vi "Keyence LJ-X8000A Read Profiles(for High Speed Data Communication).vi"() -> ()   [LabVIEW 2010]
doc: "This example mainly indicates how to acquire profiles from controllers by using <B>Read Profiles (for High-Speed Communication)</B> VI via high-speed communication."
uses:
  KEYENCE LJ-X8000A.lvlib
  Public/Clusters/Ethernet Config.ctl
  Public/Clusters/High-Speed Comm Start Req.ctl
  Public/Constants/High-Speed Comm Start Pos.ctl
  Public/Constants/High-Speed Receive Ratio.ctl
  Public/Clusters/Profile Info.ctl
panel:
  out "error out":errorcluster
  out "Comm":bool
  out "Monitoring":bool
  out "Timeout Cnt":u32
  out "Height Image":dbl[][](graph)
  out "Read Cnt":u32
  out "Notify":u32
  out "Buf Usage Rate":u32
  out "Profile Info":T1
  in  "Start Req":T2={"High-Speed Comm Start Pos"=2, "Read Profile Cnt"=1000, "High-Speed Receive Ratio"=16} {"High-Speed Receive Ratio" items=["LOWEST"=0, "LOW"=16, "MIDDLE"=17, "HIGH"=18, "HIGHEST"=32]; "High-Speed Comm Start Pos" items=["SEND COMPLETE POS", "OLDEST", "NEXT"]}
  in  "Port No":u16=24692
  in  "Stop Monitoring":bool
  in  "Start Monitoring":bool
  in  "Stop High Speed Comm":bool
  in  "Start High Speed Comm":bool
  in  "Stop VI":bool
  in  "Ethernet Config":T5={"IP Address"=[192, 168, 0, 1], "Port No"=24691}
  # "Read Profiles Start/Stop"
  # "High Speed Data Communication Start/Stop"
  # "Communication Configuration"
  # "Output from Read Profiles VI"
  # "Communication Configuration\nfor High Speed Communication"
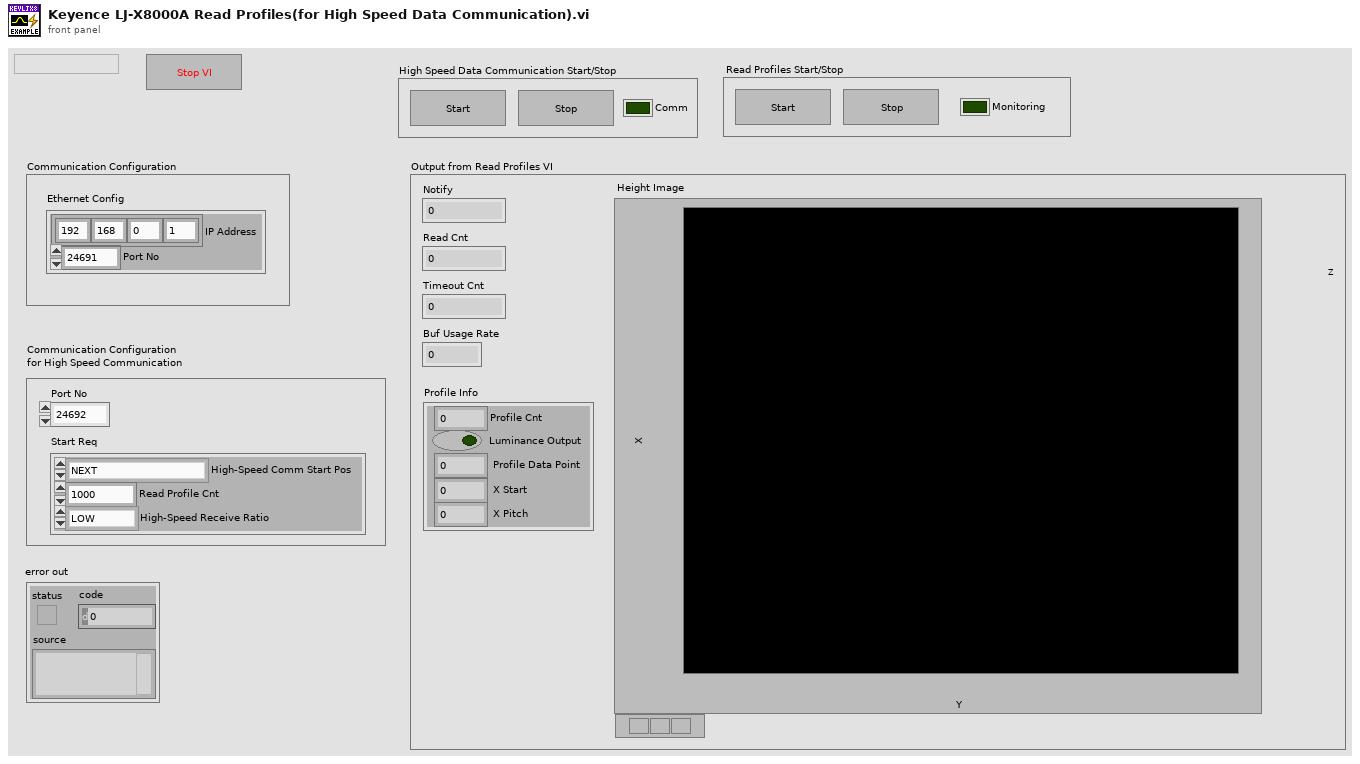
[diagram p1: front panel]
types:
  T1 = typedef "KEYENCE LJ-X8000A.lvlib/Profile Info.ctl" = cluster{"Profile Cnt":u8, "Luminance Output":bool, " Profile Data Point":u16, " X Start":i32, " X Pitch":i32}
  T2 = typedef "KEYENCE LJ-X8000A.lvlib/High-Speed Comm Start Req.ctl" = cluster{"High-Speed Comm Start Pos":T3, "Read Profile Cnt":u32, "High-Speed Receive Ratio":T4}
  T3 = typedef "KEYENCE LJ-X8000A.lvlib/High-Speed Comm Start Pos.ctl" = u8
  T4 = typedef "KEYENCE LJ-X8000A.lvlib/High-Speed Receive Ratio.ctl" = u8
  T5 = typedef "KEYENCE LJ-X8000A.lvlib/Ethernet Config.ctl" = cluster{"IP Address":u8[], "Port No":u16}
  T6 = enum8{"Enabled", "Disabled", "Disabled and Grayed Out"}
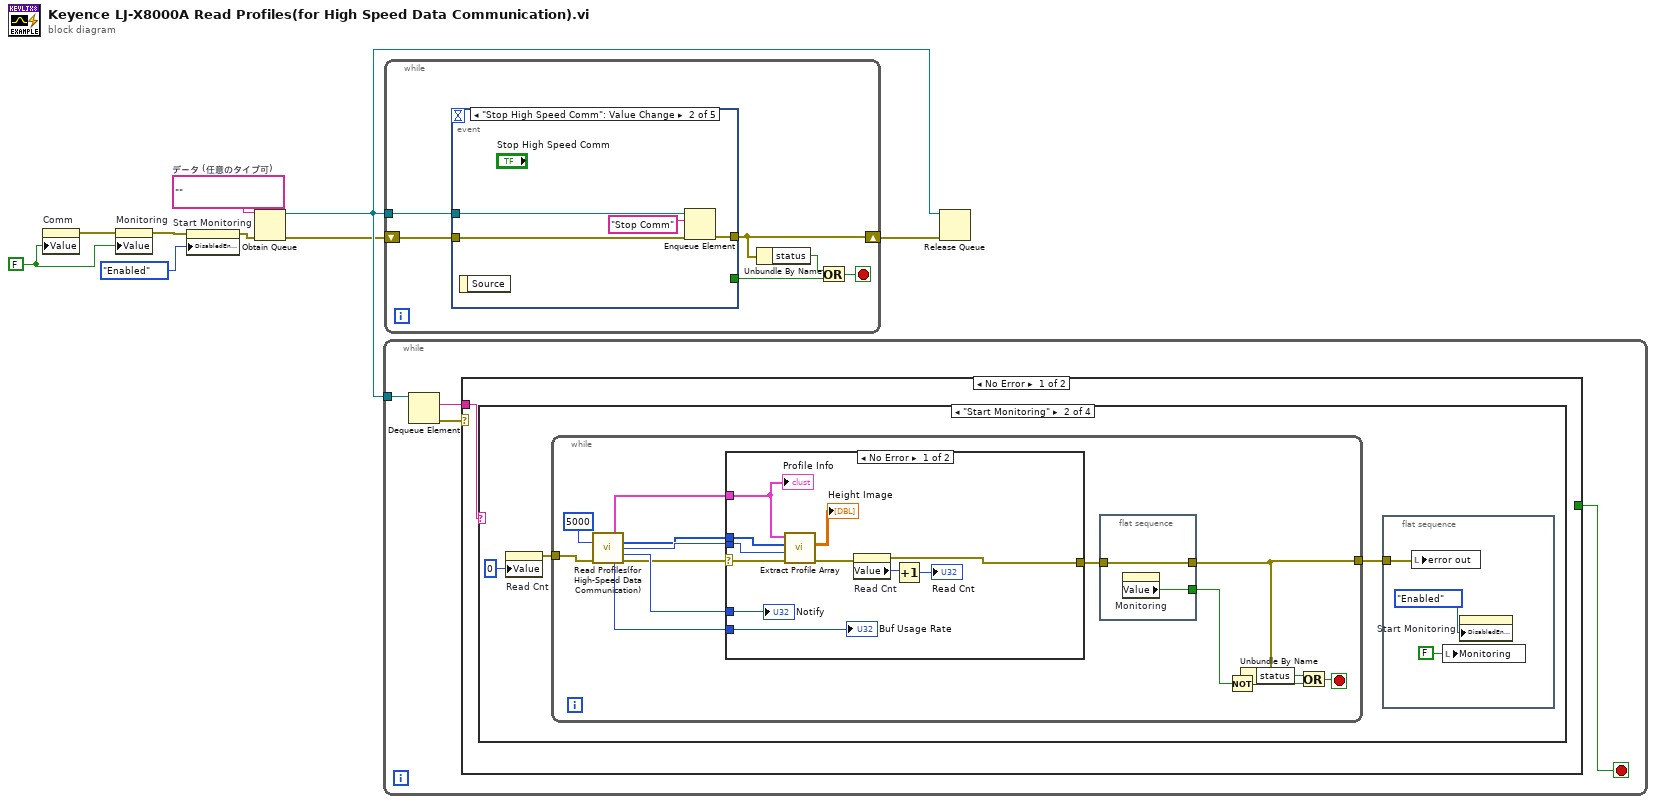
[diagram p0: block diagram]
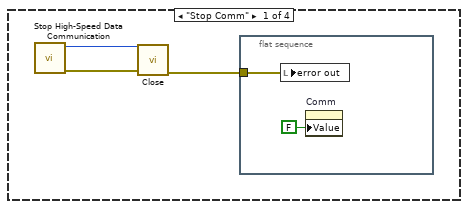
[diagram p2: hidden frame]
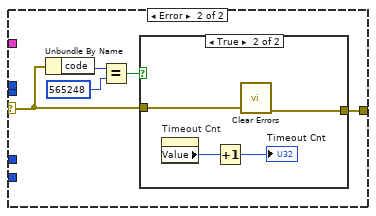
[diagram p3: hidden frame]
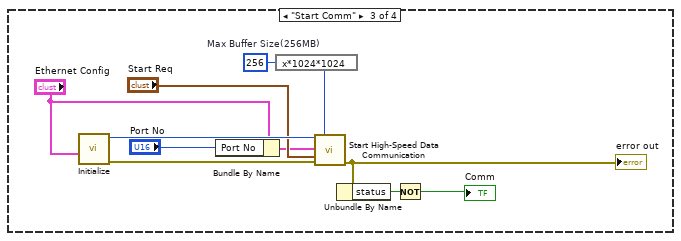
[diagram p5: hidden frame]
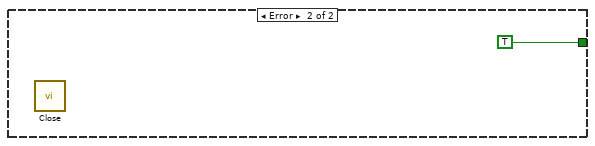
[diagram p7: hidden frame]
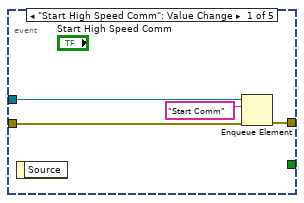
[diagram p8: hidden frame]
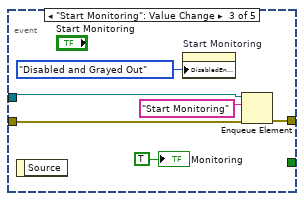
[diagram p9: hidden frame]
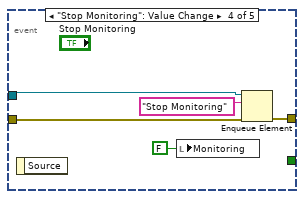
[diagram p10: hidden frame]
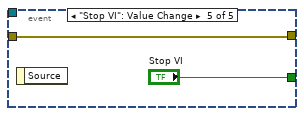
[diagram p11: hidden frame]
diagram:
  w5 = FALSE ("Monitoring")
  w7 = ""  # データ (任意のタイプ可)
  n1 = property on="Comm" class="Bool (strict)"("Value"=w5) -> (error out=w6:errorcluster)  [unwired: 2 in, 1 out]
  n2 = property on="Monitoring" class="Bool (strict)"(error in=w6, "Value"=w5) -> (error out=w4:errorcluster)  [unwired: 1 in, 1 out]
  n3 = property on="Start Monitoring" class="Bool"(error in=w4, "DisabledEnum"=T6."Enabled" ("–³Œø")) -> (error out=w2:errorcluster)  [unwired: 1 in, 1 out]
  n4 = Obtain Queue(element data type=w7, error in (no error)=w2) -> (queue out=w8:refnum<queue>, error out=w3:errorcluster)  [unwired: 3 in, 1 out]
  n5 = while {
    tunnel: w8 -> [w13]
    stop <- w10 stop-if-true
    n6 = Dequeue Element(queue=w13) -> (element=w11:string, error out=w12:errorcluster)  [unwired: 2 in, 2 out]
    n7 = case shown="No Error" w12 {
      tunnel: w11 -> [w14 _]
      tunnel: [_ TRUE] -> w10
      frame No Error {
        n8 = case shown="\"Start Monitoring\"" w14 {
          frame "Stop Comm" {
            n9 = call "Stop High-Speed Data Communication.vi"() -> ("error out"=w17:errorcluster, "Device ID out"=w16:i32)  [unwired: 10 in]
            n10 = call "Close.vi"("error in (no error)"=w17, "Device ID (0)"=w16) -> ("error out"=w15:errorcluster)  [unwired: 8 in, 1 out]
            n11 = flat-sequence {
              tunnel: w15 -> [w19]
              frame #0 {
                n12 = local write "error out"(w19) -> ()
                n13 = property on="Comm" class="Bool (strict)"("Value"=FALSE ("Comm")) -> ()  [unwired: 2 in, 2 out]
              }
            }
          }
          frame "Start Monitoring" {
            n14 = property on="Read Cnt" class="DigNum (strict)"("Value"=u32 0 ("Read Cnt")) -> (error out=w21:errorcluster)  [unwired: 2 in, 1 out]
            n15 = while {
              tunnel: w21 -> [w34]
              tunnel: [w29] -> w22
              stop <- w31 stop-if-true
              n16 = call "Read Profiles(for High-Speed Data Communication).vi"("Timeout"=u32 5000, "error in (no error)"=w34) -> ("Profile Info"=w38:T1, "Profile Data"=w32:u32[], "Rsp Profile Cnt"=w35:u32, "Notify"=w36:u32, "Buf Usage Rate"=w39:u32, "error out"=w27:errorcluster)  [unwired: 7 in, 1 out]
              n17 = case shown="No Error" w27 {
                selector: w27 -> [w47 w57]
                tunnel: w39 -> [w52 _]
                tunnel: w38 -> [w46 _]
                tunnel: w36 -> [w51 _]
                tunnel: w35 -> [w44 _]
                tunnel: [w48 w56] -> w30
                tunnel: w32 -> [w45 _]
                frame No Error {
                  n18 = call "Extract Profile Array.vi"("error in (no error)"=w47, "Profile Cnt"=w44, "Profile Data"=w45, "Profile Info"=w46) -> ("error out"=w43:errorcluster, "Height Profile Array"=→"Height Image":dbl[][])  [unwired: 4 in, 2 out]
                  n19 = property on="Read Cnt" class="DigNum (strict)"(error in=w43) -> (error out=w48:errorcluster, "Value"=w50:u32)  [unwired: 1 in, 1 out]
                  n20 = Increment(x=w50) -> (x+1=→"Read Cnt":u32)
                  "Buf Usage Rate" <- w52
                  "Profile Info" <- w46
                  "Notify" <- w51
                }
                frame Error {
                  n21 = Unbundle By Name(w57) -> ("code"=w55:i32)
                  n22 = Equal?(x=w55, y=565248) -> (x = y?=w53:bool)
                  n23 = case shown="True" w53 {
                    tunnel: w57 -> [w58 w62]
                    tunnel: [w58 w61] -> w56
                    frame False {
                    }
                    frame True {
                      n24 = property on="Timeout Cnt" class="DigNum (strict)"() -> ("Value"=w60:u32)  [unwired: 2 in, 2 out]
                      n25 = Increment(x=w60) -> (x+1=→"Timeout Cnt":u32)
                      n26 = call <vilib>:"Clear Errors.vi"("error in (no error)"=w62) -> ("error out"=w61:errorcluster)  [unwired: 5 in, 1 out]
                    }
                  }
                }
              }
              n27 = flat-sequence {
                tunnel: w30 -> [w41]
                tunnel: [w41] -> w29
                tunnel: [w40] -> w28
                frame #0 {
                  n28 = property on="Monitoring" class="Bool (strict)"() -> ("Value"=w40:bool)  [unwired: 2 in, 2 out]
                }
              }
              n29 = Not(x=w28) -> (.not. x?=w33:bool)
              n30 = Unbundle By Name(w29) -> ("status"=w26:bool)
              n31 = Or(x=w26, y=w33) -> (x .or. y?=w31:bool)
            }
            n32 = flat-sequence {
              tunnel: w22 -> [w23]
              frame #0 {
                n33 = local write "error out"(w23) -> ()
                n34 = local write "Monitoring"(FALSE ("Monitoring")) -> ()
                n35 = property on="Start Monitoring" class="Bool"("DisabledEnum"=T6."Enabled" ("–³Œø")) -> ()  [unwired: 2 in, 2 out]
              }
            }
          }
          frame "Start Comm" {
            w64 = u32 256  # Max Buffer Size(256MB)
            n36 = call "Initialize.vi"("Ethernet Config"="Ethernet Config") -> ("error out"=w66:errorcluster, "Device ID out"=w73:i32)  [unwired: 9 in]
            n37 = Bundle By Name(cluster="Ethernet Config", "Port No"="Port No") -> (w69:T5)
            n38 = expression code="x*1024*1024"(w64) -> (w68:u32)
            n39 = call "Start High-Speed Data Communication.vi"("Device ID"=w73, "Max Buffer Size"=w68, "Ethernet Config"=w69, "Start Req"="Start Req", "error in (no error)"=w66) -> ("error out"=w65:errorcluster)  [unwired: 9 in, 1 out]
            "error out" <- w65
            n40 = Unbundle By Name(w65) -> ("status"=w63:bool)
            n41 = Not(x=w63) -> (.not. x?=→"Comm":bool)
          }
          frame Default {
          }
        }
      }
      frame Error {
        n42 = call "Close.vi"() -> ()  [unwired: 10 in, 2 out]
      }
    }
  }
  n43 = while {
    shift-right: [w76] -> w9
    shift-left: w3 -> [w79]
    tunnel: w8 -> [w80]
    stop <- w77 stop-if-true
    n44 = event shown="[1] \"Stop High Speed Comm\": Value Change" {
      selector: _ -> [_ _ _ _ _]
      dyn-events: _ -> [_ _ _ _ _]
      timeout: _ -> [_ _ _ _ _]
      tunnel: w80 -> [w84 w88 w90 w95 _]
      tunnel: w79 -> [w83 w87 w94 w99 w101]
      tunnel: [w82 w86 w93 w98 w101] -> w76
      tunnel: [_ _ _ _ "Stop VI"] -> w78
      event "Start High Speed Comm": Value Change {
        n45 = event-data() -> ()  [unwired: 1 in, 1 out]
        n46 = Enqueue Element(queue=w84, element="Start Comm", error in (no error)=w83) -> (error out=w82:errorcluster)  [unwired: 1 in, 2 out]
      }
      event "Stop High Speed Comm": Value Change {
        n47 = event-data() -> ()  [unwired: 1 in, 1 out]
        n48 = Enqueue Element(queue=w88, element="Stop Comm", error in (no error)=w87) -> (error out=w86:errorcluster)  [unwired: 1 in, 2 out]
      }
      event "Start Monitoring": Value Change {
        n49 = event-data() -> ()  [unwired: 1 in, 1 out]
        n50 = property on="Start Monitoring" class="Bool"("DisabledEnum"=T6."Disabled and Grayed Out" ("–³Œø")) -> ()  [unwired: 2 in, 2 out]
        n51 = Enqueue Element(queue=w90, element="Start Monitoring", error in (no error)=w94) -> (error out=w93:errorcluster)  [unwired: 1 in, 2 out]
        "Monitoring" <- TRUE ("Monitoring")
      }
      event "Stop Monitoring": Value Change {
        n52 = event-data() -> ()  [unwired: 1 in, 1 out]
        n53 = local write "Monitoring"(FALSE ("Monitoring")) -> ()
        n54 = Enqueue Element(queue=w95, element="Stop Monitoring", error in (no error)=w99) -> (error out=w98:errorcluster)  [unwired: 1 in, 2 out]
      }
      event "Stop VI": Value Change {
        n55 = event-data() -> ()  [unwired: 1 in, 1 out]
      }
    }
    n56 = Unbundle By Name(w76) -> ("status"=w75:bool)
    n57 = Or(x=w75, y=w78) -> (x .or. y?=w77:bool)
  }
  n58 = Release Queue(queue=w8, error in (no error)=w9) -> ()  [unwired: 1 in, 3 out]
